vi "FindEmptySubpanel.vi"(8 "error in (no error)":errorcluster, 10 "Match Index":i32, 11 "SMO.UI.MAUI in":refnum<class "SMO.UI.MAUI.lvclass">) -> (0 "error out":errorcluster, 1 "Subpanel Index":i32, 2 "Ring Control":refnum<vi>, 3 "SMO.UI.MAUI out":refnum<class "SMO.UI.MAUI.lvclass">, 4 "Empty Subpanel Exists?":bool)   [LabVIEW 2020, in "SMO.UI.MAUI.lvclass"]
uses:
  SMO.UI.MAUI.lvclass
  SMO.UI.MAUI.lvclass/SMO.UI.MAUI.ctl
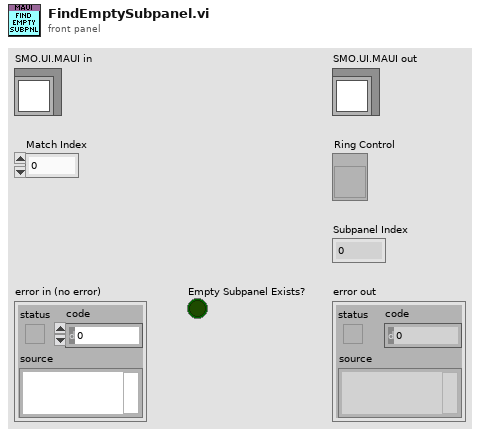
[diagram p1: front panel]
types:
  T1 = typedef "SMO.UI.MAUI.lvclass/PanelData.ctl" = cluster{"SubPanel":refnum<vi>, "Ring":refnum<vi>, "Active":i32}
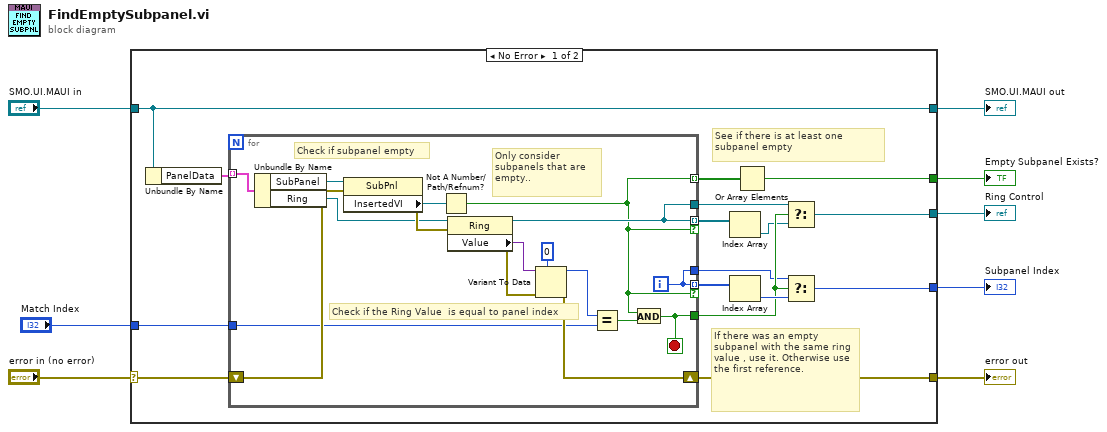
[diagram p0: block diagram]
diagram:
  n1 = case shown="No Error" "error in (no error)" {
    selector: "error in (no error)" -> [w22 w43]
    tunnel: [w21 w43] -> w7
    tunnel: [w24 w42] -> w5
    tunnel: "SMO.UI.MAUI in" -> [w24 w42]
    tunnel: "Match Index" -> [w20 _]
    tunnel: [w11 _] -> w3
    tunnel: [w10 _] -> w2
    tunnel: [w9 _] -> w1
    frame No Error {
      # "See if there is at least one subpanel empty"
      # "If there was an empty subpanel with the same ring value , use it. Otherwise use the first reference."
      n2 = Unbundle By Name(w24) -> ("PanelData"=w23:T1[])
      n3 = for {
        tunnel: w23 -> [w41] mode=indexing
        shift-right: [w35] -> w21
        shift-left: w22 -> [w37]
        tunnel: [w32] -> w16
        tunnel: [w27] -> w18 mode=indexing if=w25
        tunnel: w20 -> [w30]
        tunnel: [w28] -> w19 mode=indexing if=w25
        tunnel: [w28] -> w15
        tunnel: [w27] -> w13
        tunnel: [w25] -> w12 mode=indexing
        i -> [w27]
        stop <- w32 stop-if-true
        # "Only consider subpanels that are empty.."
        # "Check if the Ring Value  is equal to panel index"
        # "Check if subpanel empty"
        n4 = Unbundle By Name(w41) -> ("SubPanel"=w40:refnum<vi>, "Ring"=w29:refnum<vi>)
        n5 = property class="SubPnl"(reference=w40, error in=w37) -> (error out=w38:errorcluster, "InsertedVI"=w39:refnum<vi>)  [unwired: 1 out]
        n6 = Not A Number/Path/Refnum?(number/path/refnum=w39) -> (NaN/Path/Refnum?=w25:bool)
        n7 = property class="Ring"(reference=w29, error in=w38) -> (reference out=w28:refnum<vi>, error out=w36:errorcluster, "Value"=w26:variant)
        n8 = Variant To Data(error in=w36, type=0, Variant=w26) -> (data=w31:i32, error out=w35:errorcluster)
        n9 = Equal?(x=w31, y=w30) -> (x = y?=w33:bool)
        n10 = And(x=w25, y=w33) -> (x .and. y?=w32:bool)
      }
      n11 = Index Array(array=w19) -> (element=w14:refnum<vi>)  [unwired: 1 in]
      n12 = Index Array(array=w18) -> (element=w17:i32)  [unwired: 1 in]
      n13 = Or Array Elements(Boolean array=w12) -> (logical OR=w11:bool)
      n14 = Select(t=w15, s=w16, f=w14) -> (s? t:f=w9:refnum<vi>)
      n15 = Select(t=w13, s=w16, f=w17) -> (s? t:f=w10:i32)
    }
    frame Error {
    }
  }
  "error out" <- w7
  "SMO.UI.MAUI out" <- w5
  "Empty Subpanel Exists?" <- w3
  "Ring Control" <- w1
  "Subpanel Index" <- w2
